vi "Get Gyro.vi"() -> (3 "Angle":dbl)   [LabVIEW 2016]
uses:
  Robot Code/Robot Global Data.vi
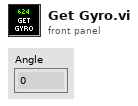
[diagram p1: front panel]
types:
  T1 = typedef "WPI_GyroDevRef.ctl" = cluster{"DevStatus":errorcluster, "Analog Channel":T2, "Offset":dbl, "Gain (VoltsPerDegree/Second)":dbl, "Gyro Type":enum16{"Analog", "XRS450"}, "Handle":i32, "SPI Bus":T3, "Device Found":bool, "Sample Rate":dbl, "Calibrate On Open":bool}
  T2 = typedef "FPGA_AIChannel.ctl" = enum8{"AI 0", "AI 1", "AI 2", "AI 3", "AI MXP 0", "AI MXP 1", "AI MXP 2", "AI MXP 3", "Invalid"}
  T3 = typedef "spi_bus.ctl" = enum16{"SPI On-Board, CS0", "SPI On-Board, CS1", "SPI On-Board, CS2", "SPI On-Board, CS3", "SPI MXP", "Invalid"}
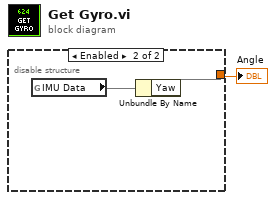
[diagram p0: block diagram]
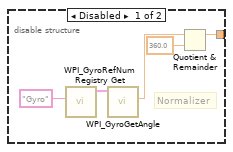
[diagram p2: hidden frame]
diagram:
  n1 = disable-structure shown="Enabled" {
    disable-tunnel: [w2 w7] -> w1
    frame Disabled {
      # "Normalizer"
      n2 = call <vilib>:"WPI_GyroRefNum Registry Get.vi"("refnum name"="Gyro") -> ("GyroDevRef"=w5:T1)  [unwired: 9 in, 1 out]
      n3 = call <vilib>:"WPI_GyroGetAngle.vi"("GyroDevRef"=w5) -> ("Angle"=w4:dbl)  [unwired: 6 in, 4 out]
      n4 = Quotient & Remainder(x=w4, y=360.0) -> (x-y*floor(x/y)=w2:dbl)  [unwired: 1 out]
    }
    frame Enabled {
      n5 = global read "Robot Global Data.vi" "IMU Data"() -> (w8)
      n6 = Unbundle By Name(w8) -> ("Yaw"=w7)
    }
  }
  "Angle" <- w1
